vi "Copy Gantry Data.vi"(8 "error in":errorcluster, 10 "Gantry Source":refnum<class "Gantry.lvclass">, 11 "Gantry Dest":refnum<class "Gantry.lvclass">) -> (0 "error out":errorcluster, 3 "Gantry Result":refnum<class "Gantry.lvclass">)   [LabVIEW 2024, in "Gantry.lvclass"]
uses:
  Gantry.lvclass
  Gantry.lvclass/Gantry.ctl
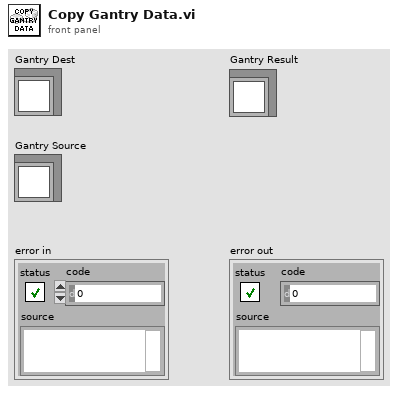
[diagram p1: front panel]
types:
  T1 = typedef "Virtual Modes.ctl" = enum16{"Nonvirtual", "Virtual"}
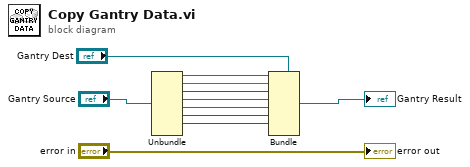
[diagram p0: block diagram]
diagram:
  n1 = Unbundle("Gantry Source") -> (w8:refnum<k24>, w7:string, w6:T1, w5:refnum<class "Vec3d.lvclass">, w4:refnum<class "FlexWorktable.lvclass">, w3:variant, w2:variant)  [unwired: 1 out]
  n2 = Bundle(cluster="Gantry Dest", w8, w7, w6, w5, w4, w3, w2) -> (→"Gantry Result":refnum<class "Gantry.lvclass">)  [unwired: 1 in]
  "error out" <- "error in"
